vi "Run Radio Test.vi"(8 "error in (no error)":errorcluster, 10 "Position":u32, 11 "MTS Radio Test in":refnum<class "MTS Radio Test.lvclass">) -> (0 "error out":errorcluster, 3 "Passed":bool)   [LabVIEW 2015, in "MTS Radio Test.lvclass"]
uses:
  MTS Radio Test.lvclass
  <vilib>/Cree, Inc/Cree Test Framework/Core Launcher/Core Manager Methods -- Enum.ctl
  Common RF Tests/RF Common Tests.lvclass
  Classes/Application/Class/Application.lvclass
  Test Class/Test Class.lvclass
  Classes/Test Recipe/Class/Test Recipe.lvclass
  <vilib>/Cree, Inc/Cree Test Framework/Classes/Data/Data Repo/Class/Data Repo.lvclass
  <vilib>/Cree, Inc/Cree Test Framework/Core Launcher/Core Launcher.lvlib
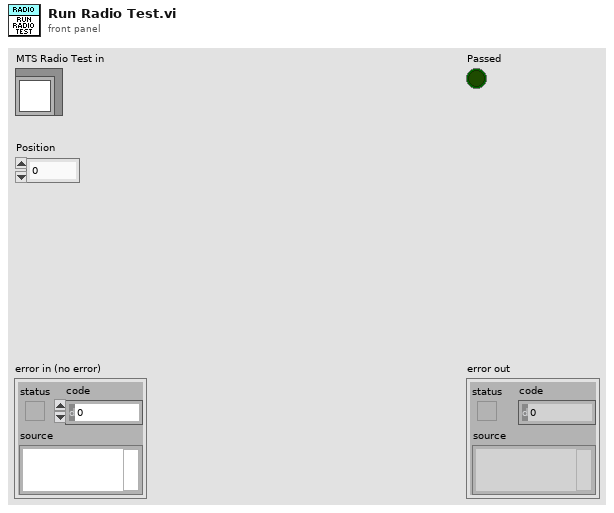
[diagram p1: front panel]
types:
  T1 = typedef "Application.lvlib/App Properties.lvclass/Class Properties -- Cluster.ctl" = cluster{"UUT Info":T2[], "Test Information":refnum<vi>, "Test Complete Event":refnum<user-event>, "Shop Floor System":refnum<class "Shop Floor System.lvclass">, "Gold Board":refnum<class "Golden Board.lvclass">, "Test Recipe":refnum<class "Test Recipe.lvclass">, "Instruments":refnum<class "Base Class.lvclass">[], "Mode":T3, "Test Results":cluster{"Pass":bool[], "Fail Codes":string[]}}
  T2 = typedef "Application.lvlib/App Properties.lvclass/UUT Reference -- Cluster.ctl" = cluster{"Serial Number Reference":refnum<vi>, "Status Message Reference":refnum<vi>}
  T3 = typedef "Application.lvlib/Application.lvclass/Op Mode -- Enum.ctl" = u16
  T4 = typedef "Core Launcher.lvlib/Core Manager Methods -- Enum.ctl" = enum16{"Spawn Objects", "Get Objects", "Destroy Objects"}
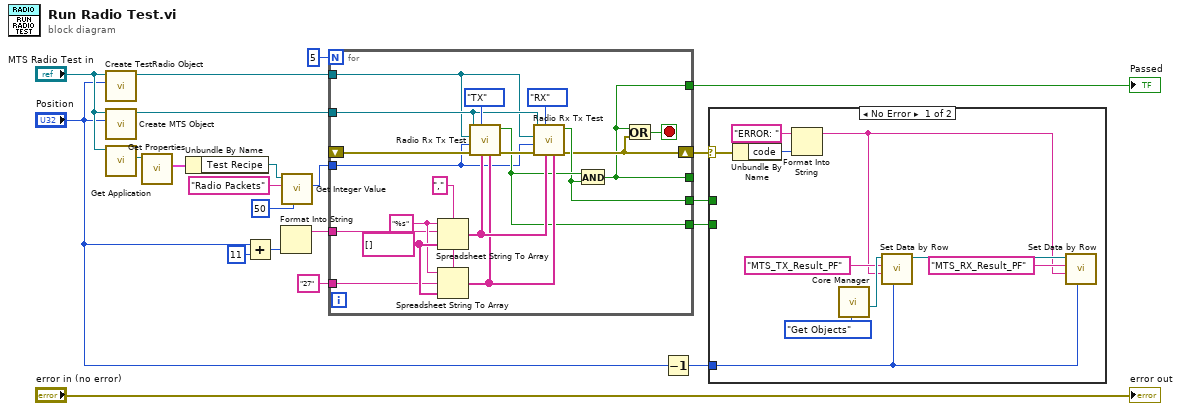
[diagram p0: block diagram]
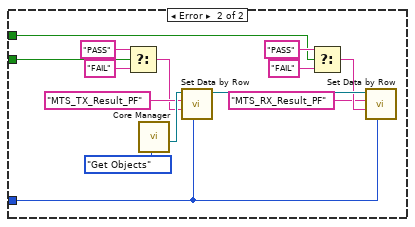
[diagram p2: hidden frame]
diagram:
  n1 = call "Create TestRadio Object.vi"("Position"="Position", "MTS Radio Test in"="MTS Radio Test in") -> ("Test Radio out"=w19:refnum<class "SC Manufacturing Test.lvclass">)  [unwired: 8 in, 1 out]
  n2 = call "Create MTS Object.vi"("Position"="Position", "RF Common Tests in"="MTS Radio Test in") -> ("SC Manufacturing Test out"=w20:refnum<class "SC Manufacturing Test.lvclass">)  [unwired: 8 in, 1 out]
  n3 = call "Get Application.vi"("Test Class in"="MTS Radio Test in") -> ("Application.lvlib:Application.lvclass"=w13:refnum<class "Application.lvclass">)  [unwired: 9 in, 1 out]
  n4 = call "Get Properties.vi"("Acrobat Template in"=w13) -> ("Class Properties"=w14:T1)  [unwired: 8 in, 2 out]
  n5 = Unbundle By Name(w14) -> ("Test Recipe"=w11:refnum<class "Test Recipe.lvclass">)
  n6 = Add(x="Position", y=u32 11) -> (x+y=w18:u32)
  n7 = Format Into String(w18) -> (resulting string=w15:string)  [unwired: 3 in, 1 out]
  n8 = call "Get Integer Value.vi"("Default Value"=u32 50, "Name"="Radio Packets", "Test Recipe in"=w11) -> ("Value"=w9:u32)  [unwired: 6 in, 2 out]
  n9 = for {
    N: 5 -> [_]
    shift-right: [w26] -> w6
    shift-left: _ -> [w34]
    tunnel: w9 -> [w24]
    tunnel: w15 -> [w36]
    tunnel: "27" ("Value") -> [w35]
    tunnel: [w27] -> w7
    tunnel: [w28] -> w8
    tunnel: [w22] -> _
    tunnel: w19 -> [w23]
    tunnel: w20 -> [w25]
    tunnel: [w22] -> w4
    stop <- w37 stop-if-true
    w38 = "%s" ("format string")
    w39 = "," ("delimiter (Tab)")
    w40 = string[] []
    n10 = Spreadsheet String To Array(delimiter (Tab)=w39, format string=w38, spreadsheet string=w36, array type (2D Dbl)=w40) -> (array=w31:string[])
    n11 = Spreadsheet String To Array(delimiter (Tab)=w39, format string=w38, spreadsheet string=w35, array type (2D Dbl)=w40) -> (array=w30:string[])
    n12 = call "Radio Rx Tx Test.vi"("Powers"=w30, "Channels"=w31, "Test to Run"=enum16{"TX", "RX"}."TX", "error in (no error)"=w34, "Packets"=w24, "Test Radio in"=w23, "SC Manufacturing Test in"=w25) -> ("error out"=w29:errorcluster, "Passed"=w28:bool)  [unwired: 3 in]
    n13 = call "Radio Rx Tx Test.vi"("Powers"=w30, "Channels"=w31, "Test to Run"=enum16{"TX", "RX"}."RX", "error in (no error)"=w29, "Packets"=w24, "Test Radio in"=w23, "SC Manufacturing Test in"=w25) -> ("error out"=w26:errorcluster, "Passed"=w27:bool)  [unwired: 3 in]
    n14 = And(x=w28, y=w27) -> (x .and. y?=w22:bool)
    n15 = Or(x=w22, y=w26) -> (x .or. y?=w37:bool)
  }
  "Passed" <- w4
  n16 = Decrement(x="Position") -> (x-1=w5:u32)
  n17 = case shown="No Error" w6 {
    selector: w6 -> [w44 _]
    tunnel: w8 -> [_ w53]
    tunnel: w7 -> [_ w52]
    tunnel: w5 -> [w45 w51]
    frame No Error {
      n18 = Unbundle By Name(w44) -> ("code"=w42:i32)
      n19 = Format Into String(initial string="ERROR: " ("Header"), w42) -> (resulting string=w41:string)  [unwired: 2 in, 1 out]
      n20 = call <vilib>:"Core Manager.vi"("Method"=Core_Manager_Methods_--_Enum."Get Objects") -> ("Data Repo"=w48:refnum<class "Data Repo.lvclass">)  [unwired: 6 in, 4 out]
      n21 = call <vilib>:"Set Data by Row.vi"("Row"=w45, "Value"=w41, "Header"="MTS_TX_Result_PF", "Acrobat Template in"=w48) -> ("Acrobat Template out"=w50:refnum<class "Data Repo.lvclass">)  [unwired: 6 in, 1 out]
      n22 = call <vilib>:"Set Data by Row.vi"("Row"=w45, "Value"=w41, "Header"="MTS_RX_Result_PF", "Acrobat Template in"=w50) -> ()  [unwired: 6 in, 2 out]
    }
    frame Error {
      n23 = Select(t="PASS" ("Header"), s=w53, f="FAIL" ("Header")) -> (s? t:f=w55:string)
      n24 = call <vilib>:"Core Manager.vi"("Method"=Core_Manager_Methods_--_Enum."Get Objects") -> ("Data Repo"=w59:refnum<class "Data Repo.lvclass">)  [unwired: 6 in, 4 out]
      n25 = call <vilib>:"Set Data by Row.vi"("Row"=w51, "Value"=w55, "Header"="MTS_TX_Result_PF", "Acrobat Template in"=w59) -> ("Acrobat Template out"=w64:refnum<class "Data Repo.lvclass">)  [unwired: 6 in, 1 out]
      n26 = Select(t="PASS" ("Header"), s=w52, f="FAIL" ("Header")) -> (s? t:f=w62:string)
      n27 = call <vilib>:"Set Data by Row.vi"("Row"=w51, "Value"=w62, "Header"="MTS_RX_Result_PF", "Acrobat Template in"=w64) -> ()  [unwired: 6 in, 2 out]
    }
  }
  "error out" <- "error in (no error)"
